vi "filtersignal.vi"(0 "Array":dbl[](array[numeric]), 1 "m":dbl, 2 "3s":dbl) -> (6 "Waveform Chart 2":i32(graph), 7 "Numeric":i32)   [LabVIEW 2014]
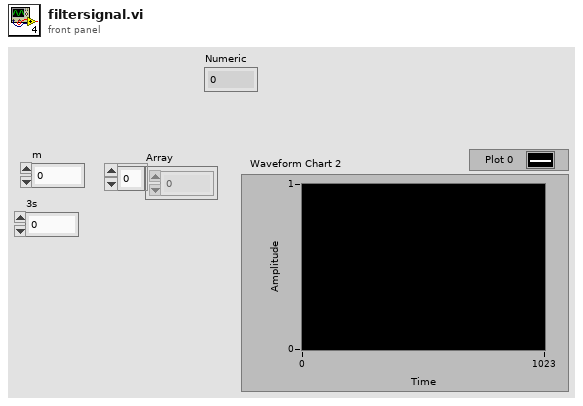
[diagram p1: front panel]
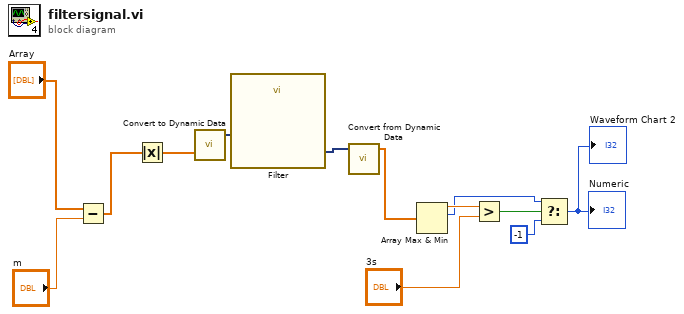
[diagram p0: block diagram]
diagram:
  n1 = Subtract(x="Array", y="m") -> (x-y=w13:dbl[])
  n2 = Absolute Value(x=w13) -> (abs(x)=w11:dbl[])
  n3 = call "Convert to Dynamic Data"("Array"=w11) -> ("Dynamic Data Type"=w9:dynamicdata)  [unwired: 3 in]
  n4 = call "Filter"("Signal"=w9) -> ("Filtered Signal"=w8:dynamicdata)  [unwired: 9 in, 1 out]
  n5 = call "Convert from Dynamic Data"("Dynamic Data Type"=w8) -> ("Array"=w7:dbl[])  [unwired: 3 in]
  n6 = Array Max & Min(array=w7) -> (max value=w6:dbl, max index (indices)=w3:i32)  [unwired: 2 out]
  n7 = Greater?(x=w6, y="3s") -> (0:w4:bool)
  n8 = Select(t=w3, s=w4, f=-1) -> (s? t:f=→"Numeric" →"Waveform Chart 2":i32)
